vi "dust_source_voltage_query.vi"(8 "error in (no error)":errorcluster) -> (0 "error out":errorcluster, 3 "high_voltage":dbl)   [LabVIEW 2013]
uses:
  <vilib>/addons/database/_DB Variant To Data/Database Variant To Data.xnode
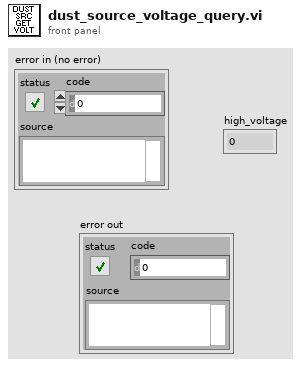
[diagram p1: front panel]
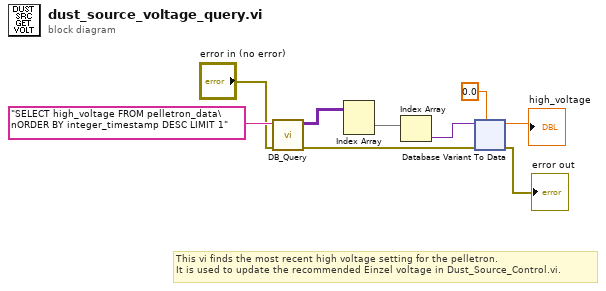
[diagram p0: block diagram]
diagram:
  # "This vi finds the most recent high voltage setting for the pelletron. \nIt is used to update the recommended Einzel voltage in Dust_Source_Control.vi."
  n1 = call "DB_Query.vi"("error in (no error)"="error in (no error)", "Parameterized Query"="SELECT high_voltage FROM pelletron_data\nORDER BY integer_timestamp DESC LIMIT 1" ("SQL query")) -> ("error out"=w7:errorcluster, "Results"=w6:variant[][])  [unwired: 7 in, 1 out]
  n2 = Index Array(array=w6) -> (element=w9:variant[])  [unwired: 2 in]
  n3 = Index Array(array=w9) -> (element=w8:variant)  [unwired: 1 in]
  n4 = xnode "Database Variant To Data"("database variant"=w8, "error in (no error)"=w7, "type"=0.0) -> ("data"=→"high_voltage":dbl, "error out"=→"error out":errorcluster)
